vi "Validate RaF Custom Device Configuration.vi"(8 "error in":errorcluster, 11 "routing and faulting in":T3 format="%.0x") -> (0 "error out":errorcluster, 2 "module connection information":T1[](array[typedef]), 3 "routing and faulting out":T3 format="%.0x")   [LabVIEW 2020, in "Routing and Faulting Scripting.lvlib"]
uses:
  Routing and Faulting Scripting.lvlib
  <vilib>/NI VeriStand/Custom Device API/Custom Device Item Ref.ctl
  Types/Module Information.ctl
  Routing and Faulting Hardware API/Types/Possible Connections for Endpoint.ctl
  <vilib>/NI VeriStand/Custom Device API/Custom Device API.lvlib
  Routing and Faulting Hardware API/Routing and Faulting Hardware API.lvlib
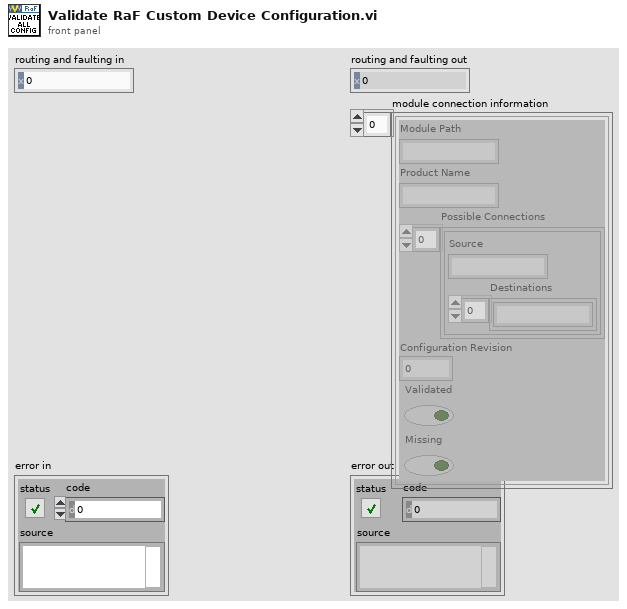
[diagram p1: front panel]
types:
  T1 = typedef "Routing and Faulting Scripting.lvlib/Module Information.ctl" = cluster{"Module Path":string, "Product Name":string, "Possible Connections":T2[], "Configuration Revision":u32, "Validated":bool, "Missing":bool}
  T2 = typedef "Routing and Faulting Hardware API.lvlib/Possible Connections for Endpoint.ctl" = cluster{"Source":string, "Destinations":string[]}
  T3 = typedef "Custom Device API.lvlib/Custom Device Item Ref.ctl" = u64
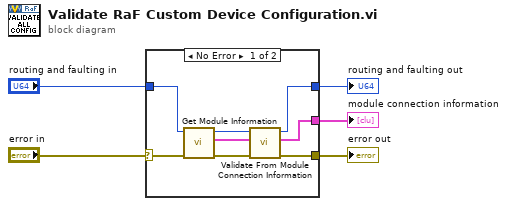
[diagram p0: block diagram]
diagram:
  n1 = case shown="No Error" "error in" {
    selector: "error in" -> [w7 w15]
    tunnel: [w10 w15] -> w5
    tunnel: "routing and faulting in" -> [w9 w14]
    tunnel: [w8 w14] -> w3
    tunnel: [w6 _] -> w1
    frame No Error {
      n2 = call "Get Module Information.vi"("error in"=w7, "routing and faulting in"=w9) -> ("error out"=w13:errorcluster, "module information"=w12:T1[], "routing and faulting out"=w11:T3)  [unwired: 7 in]
      n3 = call "Validate From Module Connection Information.vi"("error in"=w13, "module connection information in"=w12, "routing and faulting in"=w11) -> ("error out"=w10:errorcluster, "module connection information out"=w6:T1[], "routing and faulting out"=w8:T3)  [unwired: 6 in]
    }
    frame Error {
    }
  }
  "routing and faulting out" <- w3
  "error out" <- w5
  "module connection information" <- w1
